vi "Display Alarm Array.vi"() -> ()   [LabVIEW 2018, in "Dynamic Shared Variables.lvlib"]
uses:
  Dynamic Shared Variables.lvlib
  Base Tag Alarm Cluster.ctl
  Alarm Cluster.ctl
panel:
  out "blink?":bool
  out "Alarm Cluster":T1={"Color Box"=0, "Name"="", "Ack"=FALSE, "Alarm"={"alarm URL"="", "set time"=timestamp(3634824639.8324924 s since 1904-01-01), "set user"="(Nobody)", "ack time"=timestamp(-9223372036854775808 s since 1904-01-01), "ack user"="", "clear time"=timestamp(-9223372036854775808 s since 1904-01-01), "clear user"="", "setpoint"=30.0, "value"=22.498404260798484, "priority"=1, "alarm area"="", "alarm description"="", "ack comment"="", "event?"=FALSE, "Refnum"=216172782113783883}} {"Alarm"."value" format="%.2f"; "Alarm"."setpoint" format="%.2f"; "Alarm"."clear time" format="%<%X\n%x>T"; "Alarm"."ack time" format="%<%X\n%x>T"; "Alarm"."set time" format="%<%X\n%x>T"}
  in  "Alarms":T2[](array[typedef]) {"Alarm"."value" format="%.2f"; "Alarm"."setpoint" format="%.2f"; "Alarm"."clear time" format="%<%X\n%x>T"; "Alarm"."ack time" format="%<%X\n%x>T"; "Alarm"."set time" format="%<%X\n%x>T"}
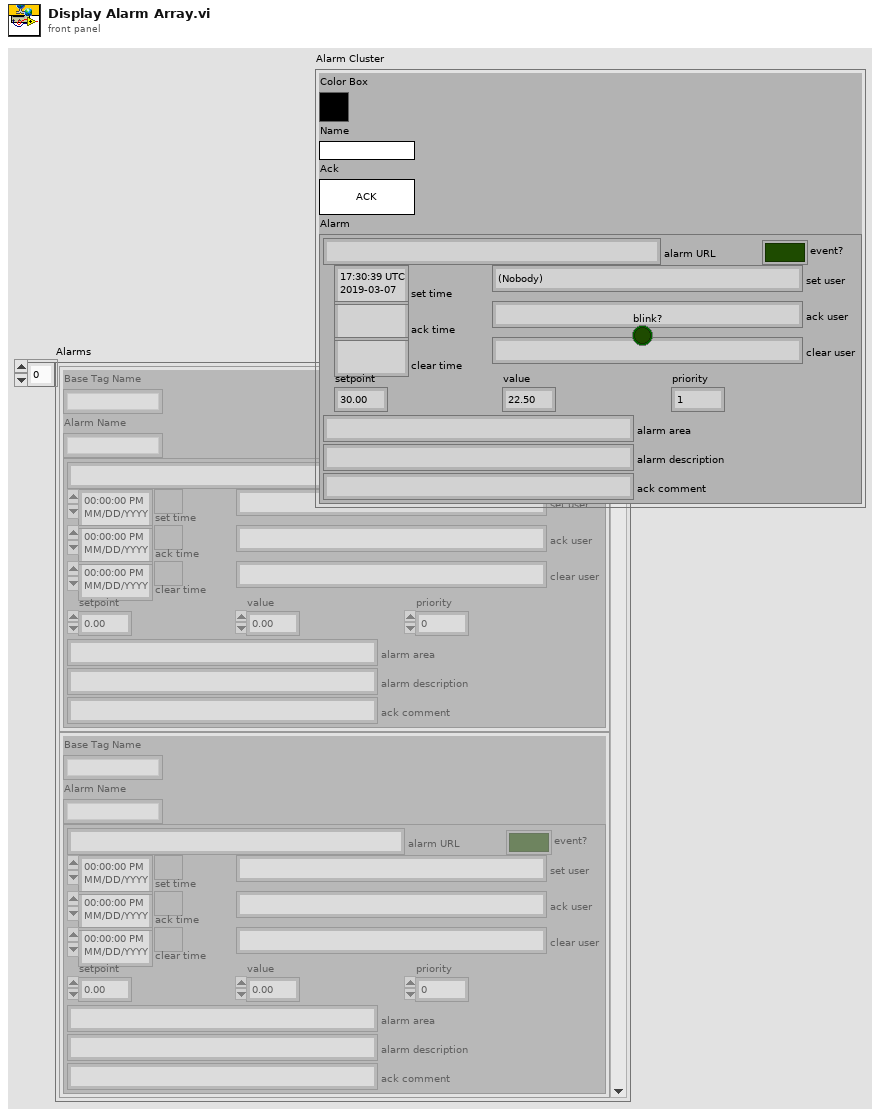
[diagram p1: front panel]
types:
  T1 = typedef "Dynamic Shared Variables.lvlib/Alarm Cluster.ctl" = cluster{"Color Box":u32, "Name":string, "Ack":bool, "Alarm":cluster{"alarm URL":string, "set time":timestamp, "set user":string, "ack time":timestamp, "ack user":string, "clear time":timestamp, "clear user":string, "setpoint":dbl, "value":dbl, "priority":u32, "alarm area":string, "alarm description":string, "ack comment":string, "event?":bool, "Refnum":u64}}
  T2 = typedef "Dynamic Shared Variables.lvlib/Base Tag Alarm Cluster.ctl" = cluster{"Base Tag Name":string, "Alarm Name":string, "Alarm":cluster{"alarm URL":string, "set time":timestamp, "set user":string, "ack time":timestamp, "ack user":string, "clear time":timestamp, "clear user":string, "setpoint":dbl, "value":dbl, "priority":u32, "alarm area":string, "alarm description":string, "ack comment":string, "event?":bool, "Refnum":u64}}
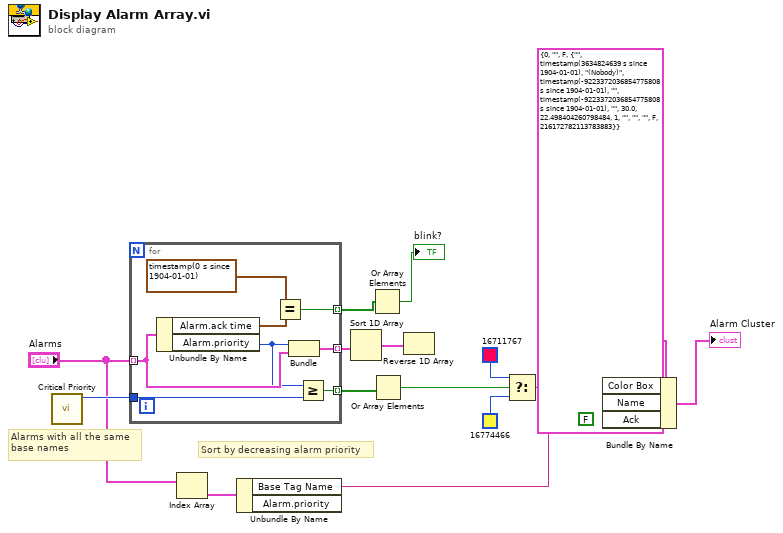
[diagram p0: block diagram]
diagram:
  # "Alarms with all the same\nbase names"
  # "Sort by decreasing alarm priority"
  n1 = call "Critical Priority.vi"() -> ("critical priority"=w12:i32)  [unwired: 11 in]
  n2 = for {
    tunnel: "Alarms" -> [w24] mode=indexing
    tunnel: [w23] -> w16 mode=indexing
    tunnel: [w20] -> w14 mode=indexing
    tunnel: w12 -> [w18]
    tunnel: [w17] -> w11 mode=indexing
    n3 = Unbundle By Name(w24) -> ("Alarm.ack time"=w21:timestamp, "Alarm.priority"=w19:u32)
    n4 = Equal?(x=timestamp(0 s since 1904-01-01) ("Alarm.ack time"), y=w21) -> (x = y?=w20:bool)
    n5 = Bundle("priority"=w19, "Cluster"=w24) -> (w23:cluster{"priority":u32, "Cluster":T2})  [unwired: 1 in]
    n6 = Greater Or Equal?(x=w19, y=w18) -> (x >= y?=w17:bool)
  }
  n7 = Index Array(array="Alarms") -> (element=w3:T2)  [unwired: 1 in]
  n8 = Unbundle By Name(w3) -> ("Base Tag Name"=w2:string)  [unwired: 1 out]
  n9 = Sort 1D Array(array=w16) -> (sorted array=w15:cluster{"priority":u32, "Cluster":T2}[])
  n10 = Or Array Elements(Boolean array=w14) -> (logical OR=→"blink?":bool)
  n11 = Or Array Elements(Boolean array=w11) -> (logical OR=w10:bool)
  n12 = Reverse 1D Array(array=w15) -> ()  [unwired: 1 out]
  n13 = Select(t=u32 16711767, s=w10, f=u32 16774466) -> (s? t:f=w5:u32)
  n14 = Bundle By Name(cluster=T1 {"Color Box"=0, "Name"="", "Ack"=FALSE, "Alarm"={"alarm URL"="", "set time"=timestamp(3634824639.8324924 s since 1904-01-01), "set user"="(Nobody)", "ack time"=timestamp(-9223372036854775808 s since 1904-01-01), "ack user"="", "clear time"=timestamp(-9223372036854775808 s since 1904-01-01), "clear user"="", "setpoint"=30.0, "value"=22.498404260798484, "priority"=1, "alarm area"="", "alarm description"="", "ack comment"="", "event?"=FALSE, "Refnum"=216172782113783883}} ("Alarm Cluster"), "Color Box"=w5, "Name"=w2, "Ack"=FALSE ("Boolean")) -> (→"Alarm Cluster":T1)
